vi "Send Async Message.vi"(4 "VI Refnum Lifetime (Destroy on Exit)":T1, 6 "Async Call Method (Call and Collect)":T2, 7 "Message Priority (Normal)":T3=enum."Normal", 8 "error in (no error)":errorcluster, 10 "Concrete Async Message":refnum<class "Async Message.lvclass">, 11 "Message Enqueuer":refnum<class "Message Enqueuer.lvclass">) -> (0 "error out":errorcluster, 2 "GUID":string, 3 "Message Enqueuer out":refnum<class "Message Enqueuer.lvclass">)   [LabVIEW 2021, in "Async Methods Actor.lvlib" / "Async Message.lvclass"]
doc: "This VI sends a concrete Async Message to an \"Async Methods Actors\" actor. \n\nWire a properly configured (see message documentation for discovering configuration options) concrete subclass of the \"Async Message\" terminal to call a specific method of a subclass of the \"Async Methods Actor\". The VI will output the GUID generated for the corresponding message sending.\n\nOptionally you can wire:\n\nan \"Async Call Method\" enumeration. This can take values \"Call and Collect\" and \"Call and Forget\". In the former case the \"Async Methods Actor\" will track the execution of the methods by waiting for their completion, in the latter case instead the actor will not wait for their completion but will just count their launch.\n\na \"VI Refnum Lifetime\" enumeration. This can take values \"Destroy on Exit\", \" Destroy on Actor Exit \", and \"Destroy on Application Exit\". This enumeration dictates the lifetime strategy adopted for the VI Refnum of the Async Method. In the first case the \"Async Methods Actor\" destroys the reference as soon as the Async Method Exits, in the second case the VI Refnums will be destroyed once the \"Async Method Actor\" exits, while in the last case, VI Refnums are never destroyed. \"Destroy on Exit\" is the default option when unwired. The motivation for this setting is related to the required lifetimes of the Refnums (e.g. notifier's references) created within the Async Method. This lifetime is the same as the VI Refnum lifetime, hence if we want they outlive the execution of the Async Method we have to set it to either \"Destroy on Actor Exit\" or \"Destroy on Application Exit\". This option applies only to Async Methods called with the \"Call and Collect\" option."
uses:
  Async Message.lvclass
  <vilib>/ActorFramework/Message Enqueuer/Message Enqueuer.lvclass
  <vilib>/ActorFramework/Message Enqueuer/Message Priority.ctl
  C:/Program Files/National Instruments/LabVIEW 2021/vi.lib/ActorFramework/Message/Message.lvclass
  Async Methods Actor/Async Call Method.ctl
  Async Methods Actor/VI Refnum Lifetime.ctl
  Async Message.lvclass/Async Message.ctl
  <vilib>/ActorFramework/Message Enqueuer/Message Enqueuer.lvclass/Message Enqueuer.ctl
  <vilib>/Utility/LVClass/Get LV Class Name.vi
  <resource>/AFDebug/Generate Trace for Message.vi
  <vilib>/ActorFramework/Message Priority Queue/Priority Enqueue.vi
  Async Methods Actor/Async Methods Actor.lvclass
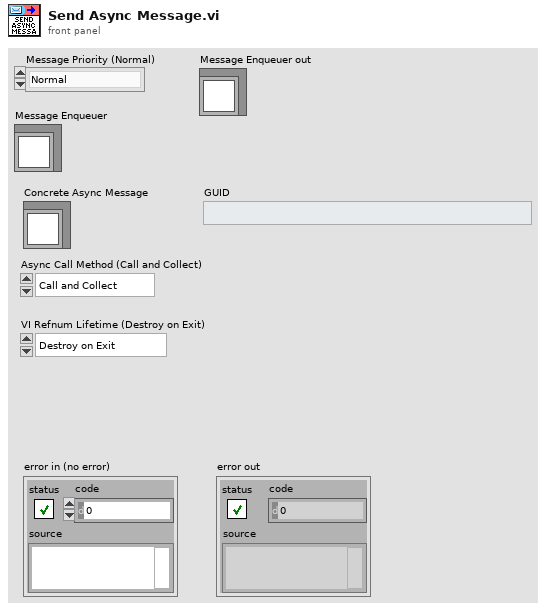
[diagram p1: front panel]
types:
  T1 = typedef "Async Methods Actor.lvlib/Async Methods Actor.lvclass/VI Refnum Lifetime.ctl" = enum16{"Destroy on Exit", "Destroy on Actor Exit", "Destroy on Application Exit"}
  T2 = typedef "Async Methods Actor.lvlib/Async Methods Actor.lvclass/Async Call Method.ctl" = enum16{"Call and Collect", "Call and Forget"}
  T3 = typedef "Actor Framework.lvlib/Message Enqueuer.lvclass/Message Priority.ctl" = enum16{"Low", "Normal", "High"}
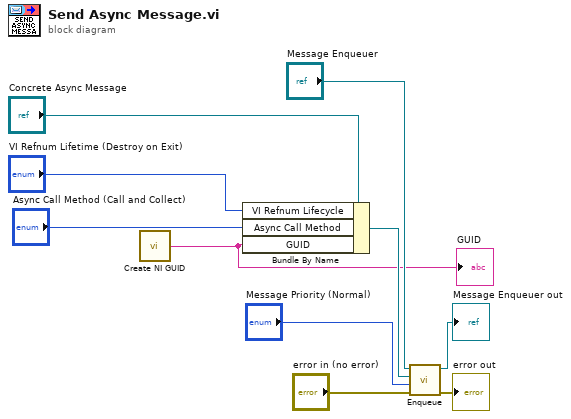
[diagram p0: block diagram]
diagram:
  n1 = call <vilib>:"Create NI GUID.vi"() -> ("NI GUID"=w2:string)
  "GUID" <- w2
  n2 = Bundle By Name(cluster="Concrete Async Message", "VI Refnum Lifecycle"="VI Refnum Lifetime (Destroy on Exit)", "Async Call Method"="Async Call Method (Call and Collect)", "GUID"=w2) -> (w5:refnum<class "Async Message.lvclass">)
  n3 = call <vilib>:"Enqueue.vi"("error in (no error)"="error in (no error)", "Message Priority (Normal)"="Message Priority (Normal)", "Message"=w5, "Message Enqueuer in"="Message Enqueuer") -> ("error out"=→"error out":errorcluster, "Message Enqueuer out"=→"Message Enqueuer out":refnum<class "Message Enqueuer.lvclass">)  [unwired: 6 in]
